vi "Page_Hardware_Write.vi"(6 "ctlReferences":T1, 8 "error in (no error)":errorcluster, 11 "Class in":refnum<class "IB_MSI.lvclass">) -> (0 "error out":errorcluster, 3 "Class out":refnum<class "IB_MSI.lvclass">)   [LabVIEW 2020, in "IB_MSI.lvclass"]
uses:
  <vilib>/AppBuilder/IB_Classes/MSI/IB_MSI.lvclass
  <resource>/Framework/Providers/Builds/Installer/Pages/controls/IB_UI_Page_Hardware_References.ctl
  <resource>/Framework/Providers/Builds/Installer/CDK_sTypeDef_HWImportOption.ctl
  <vilib>/AppBuilder/IB_Classes/MSI/IB_MSI.lvclass/IB_MSI.ctl
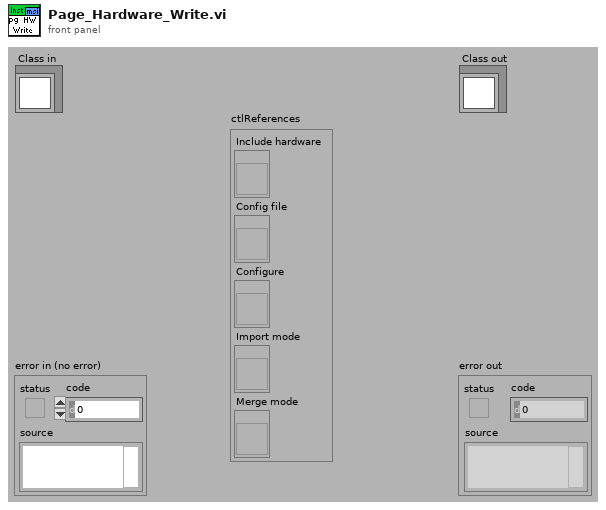
[diagram p1: front panel]
types:
  T1 = typedef "IB_UI_Page_Hardware_References.ctl" = cluster{"Include hardware":refnum<vi>, "Config file":refnum<vi>, "Configure":refnum<vi>, "Import mode":refnum<vi>, "Merge mode":refnum<vi>}
  T2 = typedef "CDK_sTypeDef_HWImportOption.ctl" = enum16{"<none>", "Merge", "Replace", "Dialog"}
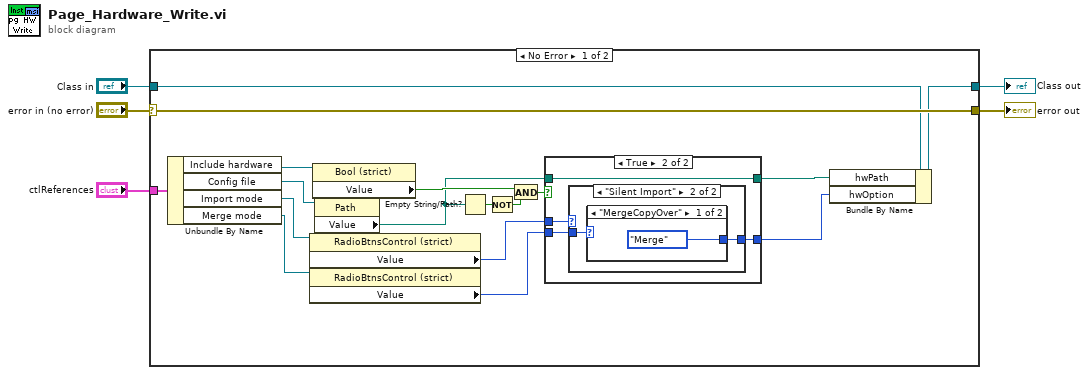
[diagram p0: block diagram]
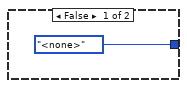
[diagram p2: hidden frame]
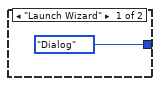
[diagram p3: hidden frame]
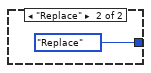
[diagram p4: hidden frame]
diagram:
  n1 = case shown="No Error" "error in (no error)" {
    selector: "error in (no error)" -> [w22 w34]
    tunnel: [w22 w34] -> w4
    tunnel: [w9 w33] -> w2
    tunnel: "Class in" -> [w10 w33]
    tunnel: "ctlReferences" -> [w15 _]
    frame No Error {
      n2 = Unbundle By Name(w15) -> ("Include hardware"=w14:refnum<vi>, "Config file"=w13:refnum<vi>, "Import mode"=w11:refnum<vi>, "Merge mode"=w12:refnum<vi>)
      n3 = property class="RadioBtnsControl (strict)"(reference=w11) -> ("Value"=w18:enum32{"Launch Wizard", "Silent Import"})  [unwired: 1 in, 2 out]
      n4 = property class="RadioBtnsControl (strict)"(reference=w12) -> ("Value"=w17:enum32{"MergeCopyOver", "Replace"})  [unwired: 1 in, 2 out]
      n5 = property class="Bool (strict)"(reference=w14) -> ("Value"=w21:bool)  [unwired: 1 in, 2 out]
      n6 = property class="Path"(reference=w13) -> ("Value"=w6:path)  [unwired: 1 in, 2 out]
      n7 = Empty String/Path?(string/path=w6) -> (empty?=w20:bool)
      n8 = Not(x=w20) -> (.not. x?=w19:bool)
      n9 = And(x=w21, y=w19) -> (x .and. y?=w16:bool)
      n10 = case shown="True" w16 {
        tunnel: w18 -> [_ w27]
        tunnel: w17 -> [_ w26]
        tunnel: [_ w25] -> w8
        tunnel: w6 -> [_ w25]
        tunnel: [CDK_sTypeDef_HWImportOption."<none>" ("HWOption") w24] -> w7
        frame False {
        }
        frame True {
          n11 = case shown="\"Silent Import\"" w27 {
            tunnel: w26 -> [_ w30]
            tunnel: [CDK_sTypeDef_HWImportOption."Dialog" ("HWOption") w29] -> w24
            frame "Launch Wizard" {
            }
            frame "Silent Import" {
              n12 = case shown="\"MergeCopyOver\"" w30 {
                tunnel: [CDK_sTypeDef_HWImportOption."Merge" ("HWOption") CDK_sTypeDef_HWImportOption."Replace" ("HWOption")] -> w29
                frame "MergeCopyOver" {
                }
                frame "Replace" {
                }
              }
            }
          }
        }
      }
      n13 = Bundle By Name(cluster=w10, "hwPath"=w8, "hwOption"=w7) -> (w9:refnum<class "IB_MSI.lvclass">)
    }
    frame Error {
    }
  }
  "error out" <- w4
  "Class out" <- w2
